vi "GetType.vi"(8 "error in (no error)":errorcluster, 11 "Configure NofBins Msg":refnum<class "Configure NofBins Msg.lvclass">) -> (0 "error out":errorcluster, 2 "Data Sample":variant, 3 "Configure NofBins Msg":refnum<class "Configure NofBins Msg.lvclass">)   [LabVIEW 2016, in "CS++MCS.lvlib" / "Configure NofBins Msg.lvclass"]
uses:
  Configure NofBins Msg.lvclass
  Configure NofBins Msg.lvclass/Configure NofBins Msg.ctl
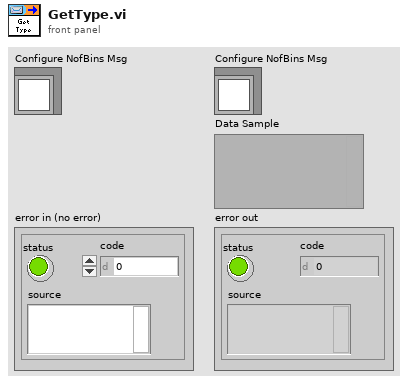
[diagram p1: front panel]
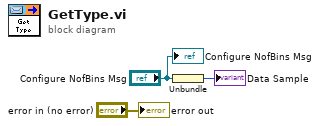
[diagram p0: block diagram]
diagram:
  n1 = Unbundle("Configure NofBins Msg") -> (→"Data Sample":i32)
  "error out" <- "error in (no error)"
  "Configure NofBins Msg" <- "Configure NofBins Msg"
